vi "dfd_Select Separator.vi"(11 "indent order":i32) -> (3 "separator":string)   [LabVIEW 2017, in "NI_DigFilter_Process.lvlib"]
uses:
  <vilib>/addons/Digital Filter Design/NI_DigFilter_Process.lvlib
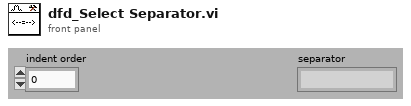
[diagram p1: front panel]
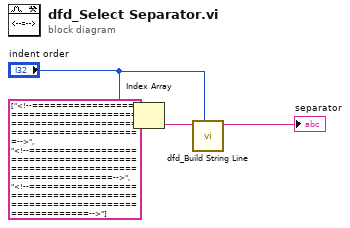
[diagram p0: block diagram]
diagram:
  n1 = Index Array(array=string[] ["<!--=================================================================================-->", "<!--=============================================================================-->", "<!--=========================================================================-->"], index="indent order") -> (element=w2:string)
  n2 = call <vilib>:"dfd_Build String Line.vi"("indent order"="indent order", "string"=w2) -> ("string line"=→"separator":string)  [unwired: 9 out]
